vi "API_DB.GetAllEmptyLocations.vi"(0 "Database in":refnum<class "Database.lvclass">, 1 "Wait (F)":bool, 5 "Table":string, 11 "error in (no error)":errorcluster, 12 "Timeout (ms)":u32) -> (4 "Database out":refnum<class "Database.lvclass">, 6 "Slot":string, 15 "error out":errorcluster)   [LabVIEW 2020, in "Database.lvclass"]
doc: "Developed by Kevin Thompson\nkevin@thompsonengineering.net\n\nCopyright 2018\nThompson Engineering, LLC"
uses:
  Database.lvclass
  DataTypes/AsynCmd_Temp01--enum.ctl
  DataTypes/GenericQuery--Cluster.ctl
  DataTypes/SQLQuery--Enum.ctl
  DataTypes/InventoryRecord--Cluster.ctl
  DataTypes/Module--Cluster.ctl
  DataTypes/LocationStatus--Enum.ctl
  Database.lvclass/Database.ctl
  DataTypes/Stocker--Enum.ctl
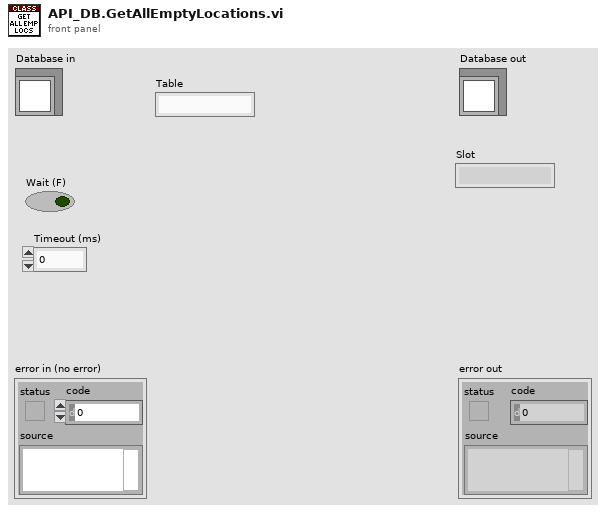
[diagram p1: front panel]
types:
  T1 = typedef "SQLQuery--Enum.ctl" = enum16{"GetInventoryRecordFromDB", "GetReticleInfoFromDB", "GetLocationStatusFromDB", "UpdateInventoryRecord", "UpdateLocationStatus", "UpdateReticleLocationStatus", "AddReticleInDB", "RemoveReticleAtLocation", "RemoveReticleUsingReticleID", "GetLocationForReticleID", "GetAllLocations", "GetAllEmptyLocations", "GetAllLocationsInStocker", "GetAllFullLocations", "GetAllFullLocationsInStocker", "GetAllDisabledLocations", "GetAllDisabledLocationsInStocker", "FindFirstSlot"}
  T2 = typedef "GenericQuery--Cluster.ctl" = cluster{"Query":T1, "Table":string, "InventoryRecord":T3}
  T3 = typedef "InventoryRecord--Cluster.ctl" = cluster{"ReticleID":string, "Stocker":T4, "Location":T5, "LocationStatus":T6, "EquipmentID":string, "LocationID":string}
  T4 = typedef "Stocker--Enum.ctl" = u16
  T5 = typedef "Module--Cluster.ctl" = cluster{"Module":u16, "Row":u16, "Column":u16}
  T6 = typedef "LocationStatus--Enum.ctl" = enum16{"Disabled/Unusable", "Full", "Empty"}
  T7 = typedef "Database.lvclass/AsynCmd_Temp01--enum.ctl" = enum16{"DB.DeleteRecord", "DB.UpdateRecord", "DB.InsertRecord", "DB.SelectRecord", "DB.ExecuteSQLCommand", "DB.FindFirstSlot", "DB.GenericSQLQuery"}
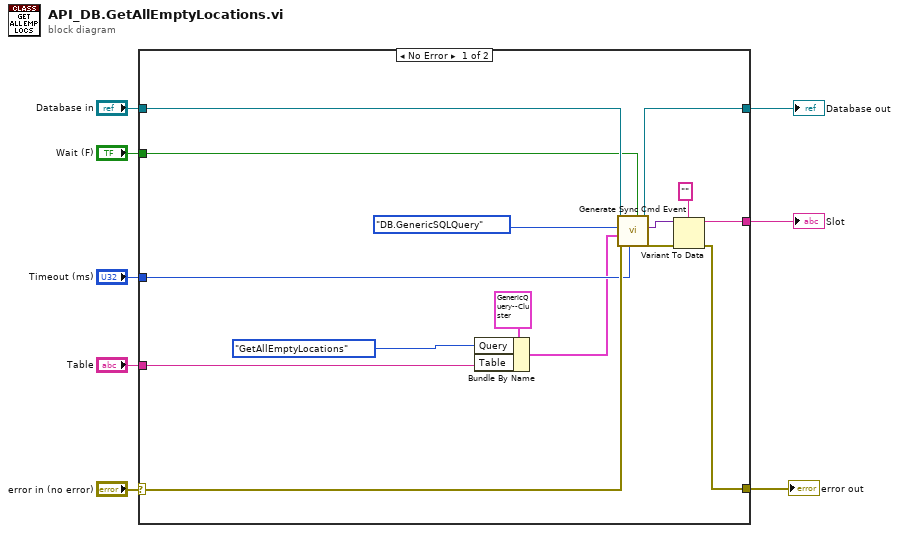
[diagram p0: block diagram]
diagram:
  n1 = case shown="No Error" "error in (no error)" {
    selector: "error in (no error)" -> [w21 w25]
    tunnel: [w16 w25] -> w7
    tunnel: [w22 w24] -> w5
    tunnel: "Database in" -> [w23 w24]
    tunnel: [w18 _] -> w2
    tunnel: "Wait (F)" -> [w15 _]
    tunnel: "Timeout (ms)" -> [w14 _]
    tunnel: "Table" -> [w9 _]
    frame No Error {
      n2 = Bundle By Name(cluster=T2 {"Query"=enum."GetInventoryRecordFromDB", "Table"="", "InventoryRecord"={"ReticleID"="", "Stocker"=0, "Location"={"Module"=0, "Row"=0, "Column"=0}, "LocationStatus"=enum."Disabled/Unusable", "EquipmentID"="", "LocationID"=""}}, "Query"=SQLQuery--Enum."GetAllEmptyLocations", "Table"=w9) -> (w10:T2)
      n3 = call "Generate Sync Cmd Event.vi"("Wait (F)"=w15, "Timeout (ms)"=w14, "error in (no error)"=w21, "vData"=w10, "AsyncCmd"=AsynCmd_Temp01--enum."DB.GenericSQLQuery", "Database in"=w23) -> ("error out"=w17:errorcluster, "Return Value"=w19:variant, "Database out"=w22:refnum<class "Database.lvclass">)  [unwired: 3 in]
      n4 = Variant To Data(error in=w17, type="", Variant=w19) -> (data=w18:string, error out=w16:errorcluster)
    }
    frame Error {
    }
  }
  "error out" <- w7
  "Database out" <- w5
  "Slot" <- w2
